vi "ExperimentalSystemDataConstant.vi"() -> (2 "Experimental System Data":T1)   [LabVIEW 2014]
uses:
  Controls/ExperimentalSystemData.ctl
panel:
  # "Bank\nVoltages"
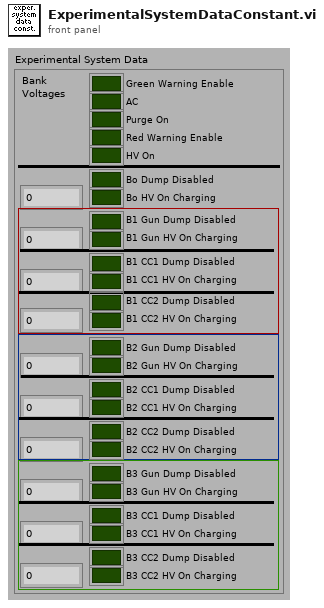
[diagram p1: front panel]
types:
  T1 = typedef "ExperimentalSystemData.ctl" = cluster{"Bo Volts":dbl, "B1 Gun":dbl, "B1 CC1":dbl, "B1 CC2":dbl, "B2 Gun":dbl, "B2 CC1":dbl, "B2 CC2":dbl, "B3 Gun":dbl, "B3 CC1":dbl, "B3 CC2":dbl, "Green Warning Enable":bool, "AC":bool, "Purge On":bool, "Red Warning Enable":bool, "HV On":bool, "Bo Dump Disabled":bool, "Bo HV On Charging":bool, "B1 Gun Dump Disabled":bool, "B1 Gun HV On Charging":bool, "B1 CC1 Dump Disabled":bool, "B1 CC1 HV On Charging":bool, "B1 CC2 Dump Disabled":bool, "B1 CC2 HV On Charging":bool, "B2 Gun Dump Disabled":bool, "B2 Gun HV On Charging":bool, "B2 CC1 Dump Disabled":bool, "B2 CC1 HV On Charging":bool, "B2 CC2 Dump Disabled":bool, "B2 CC2 HV On Charging":bool, "B3 Gun Dump Disabled":bool, "B3 Gun HV On Charging":bool, "B3 CC1 Dump Disabled":bool, "B3 CC1 HV On Charging":bool, "B3 CC2 Dump Disabled":bool, "B3 CC2 HV On Charging":bool}
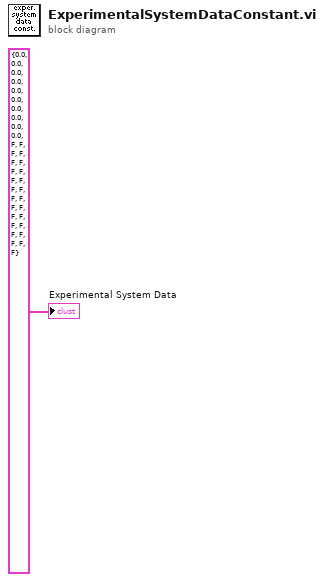
[diagram p0: block diagram]
diagram:
  "Experimental System Data" <- T1 {"Bo Volts"=0.0, "B1 Gun"=0.0, "B1 CC1"=0.0, "B1 CC2"=0.0, "B2 Gun"=0.0, "B2 CC1"=0.0, "B2 CC2"=0.0, "B3 Gun"=0.0, "B3 CC1"=0.0, "B3 CC2"=0.0, "Green Warning Enable"=FALSE, "AC"=FALSE, "Purge On"=FALSE, "Red Warning Enable"=FALSE, "HV On"=FALSE, "Bo Dump Disabled"=FALSE, "Bo HV On Charging"=FALSE, "B1 Gun Dump Disabled"=FALSE, "B1 Gun HV On Charging"=FALSE, "B1 CC1 Dump Disabled"=FALSE, "B1 CC1 HV On Charging"=FALSE, "B1 CC2 Dump Disabled"=FALSE, "B1 CC2 HV On Charging"=FALSE, "B2 Gun Dump Disabled"=FALSE, "B2 Gun HV On Charging"=FALSE, "B2 CC1 Dump Disabled"=FALSE, "B2 CC1 HV On Charging"=FALSE, "B2 CC2 Dump Disabled"=FALSE, "B2 CC2 HV On Charging"=FALSE, "B3 Gun Dump Disabled"=FALSE, "B3 Gun HV On Charging"=FALSE, "B3 CC1 Dump Disabled"=FALSE, "B3 CC1 HV On Charging"=FALSE, "B3 CC2 Dump Disabled"=FALSE, "B3 CC2 HV On Charging"=FALSE} ("Status LEDs")
